vi "LoadAndRunMaster.vi"(2 "Task":enum16{"Run", "Stop"}(ring)) -> (0 "error out":errorcluster, 1 "ROS Master":string="192.168.1.110:11311")   [LabVIEW 2012]
doc: "Loads and runs a master on a given machine"
uses:
  <userlib>/ROS for LabVIEW Software/ROS/Code/_ROSDefinition.vi
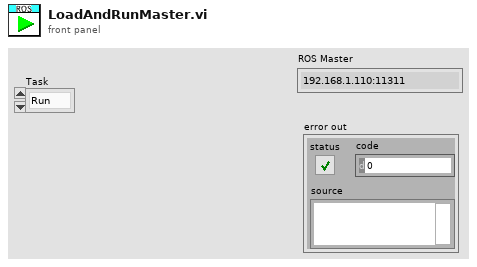
[diagram p1: front panel]
types:
  T1 = enum32{"Bad", "Idle", "Run top level", "Running"}
  T2 = enum32{"Invalid", "Standard", "Closed", "Hidden", "Minimized", "Maximized"}
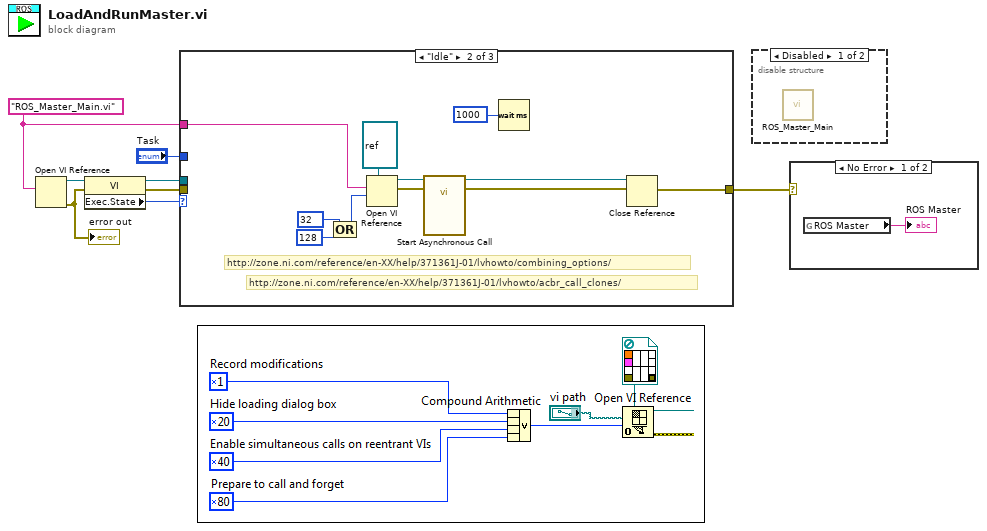
[diagram p0: block diagram]
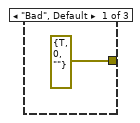
[diagram p3: hidden frame]
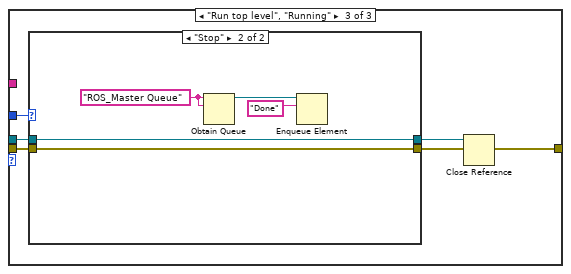
[diagram p4: hidden frame]
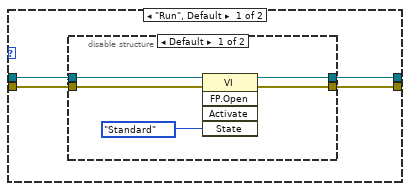
[diagram p5: hidden frame]
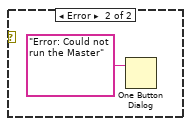
[diagram p7: hidden frame]
diagram:
  w1 = "ROS_Master_Main.vi" ("name or relative path")
  n1 = Open VI Reference(vi path=w1) -> (vi reference=w8:refnum<vi>, error out=w7:errorcluster)  [unwired: 5 in]
  "error out" <- w7
  n2 = property class="VI"(reference=w8, error in=w7) -> (reference out=w5:refnum<vi>, error out=w4:errorcluster, "Exec.State"=w6:T1)
  n3 = case shown="\"Idle\"" w6 {
    tunnel: [errorcluster {"status"=TRUE, "code"=0, "source"=""} ("error out") w10 w21] -> w3
    tunnel: w5 -> [_ _ w26]
    tunnel: w4 -> [_ _ w25]
    tunnel: "Task" -> [_ _ w24]
    tunnel: w1 -> [_ w15 _]
    frame "Bad", Default {
    }
    frame "Idle" {
      # "http://zone.ni.com/reference/en-XX/help/371361J-01/lvhowto/acbr_call_clones/"
      # "http://zone.ni.com/reference/en-XX/help/371361J-01/lvhowto/combining_options/"
      n4 = Compound Arithmetic op=OR(32, 128) -> (w19:i32)
      n5 = Open VI Reference(type specifier VI Refnum (for type only)=refnum<vi> refnum, vi path=w15, options=w19) -> (vi reference=w14:refnum<vi>, error out=w13:errorcluster)  [unwired: 3 in]
      n6 = call-by-ref "Start Asynchronous Call"(reference=w14, error in=w13) -> (reference out=w12:refnum<vi>, error out=w11:errorcluster)  [unwired: 4 in]
      n7 = Wait (ms)(milliseconds to wait=u32 1000) -> ()  [unwired: 1 out]
      n8 = Close Reference(reference=w12, error in (no error)=w11) -> (error out=w10:errorcluster)
    }
    frame "Run top level", "Running" {
      n9 = case shown="\"Stop\"" w24 {
        tunnel: [w28 w42] -> w22
        tunnel: w26 -> [w30 w38]
        tunnel: w25 -> [w29 w42]
        tunnel: [w27 w38] -> w23
        frame "Run", Default {
          n10 = disable-structure shown="Default" {
            disable-tunnel: w30 -> [w35 w37]
            disable-tunnel: w29 -> [w34 w36]
            disable-tunnel: [w32 w36] -> w28
            disable-tunnel: [w31 w37] -> w27
            frame condition #0 (active) {
              n11 = invoke class="VI" method="FP.Open"(reference=w35, error in=w34, "State"=T2."Standard") -> (reference out=w31:refnum<vi>, error out=w32:errorcluster)  [unwired: 2 in, 3 out]
            }
            frame condition #1 {
            }
          }
        }
        frame "Stop" {
          w41 = "ROS_Master Queue" ("name (unnamed)")
          n12 = Obtain Queue(name (unnamed)=w41, element data type=w41) -> (queue out=w40:refnum<queue>)  [unwired: 3 in, 2 out]
          n13 = Enqueue Element(queue=w40, element="Done") -> ()  [unwired: 2 in, 3 out]
        }
      }
      n14 = Close Reference(reference=w23, error in (no error)=w22) -> (error out=w21:errorcluster)
    }
  }
  n15 = disable-structure shown="Disabled" {
    frame Disabled {
      n16 = call <userlib>:"ROS_Master_Main.vi"() -> ()  [unwired: 4 in]
    }
    frame Enabled {
    }
  }
  n17 = case shown="No Error" w3 {
    frame No Error {
      n18 = global read "_ROSDefinition.vi" "ROS Master"() -> (→"ROS Master":string)
    }
    frame Error {
      n19 = One Button Dialog(message="Error: Could not run the Master") -> ()  [unwired: 1 in, 1 out]
    }
  }
